vi "Timing.vi"(8 "error in (no error)":errorcluster, 11 "State":T1) -> (0 "error out":errorcluster, 3 "Array":timestamp[](array[timestamp]))   [LabVIEW 2012]
uses:
  New_Framework_2013/State_Machine_Enum.ctl
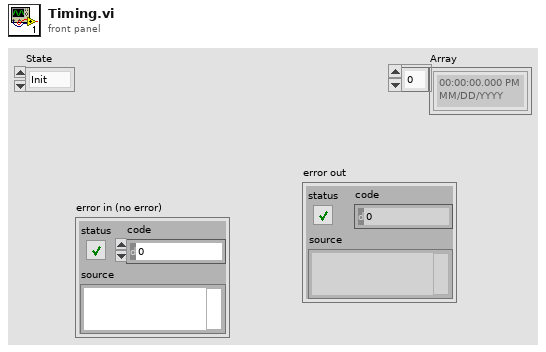
[diagram p1: front panel]
types:
  T1 = typedef "State_Machine_Enum.ctl" = enum16{"Init", "Idle", "Start", "Do", "Stop"}
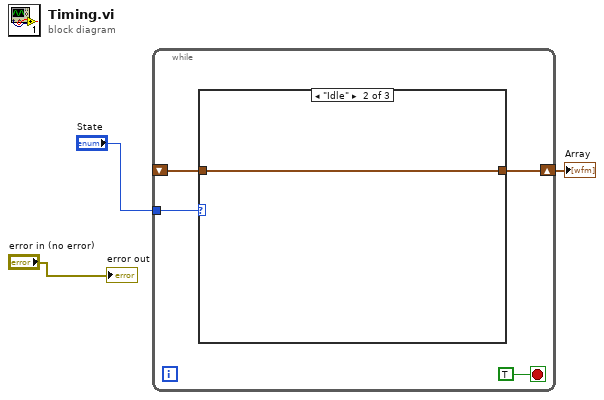
[diagram p0: block diagram]
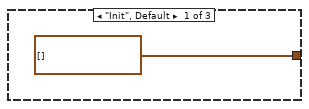
[diagram p2: hidden frame]
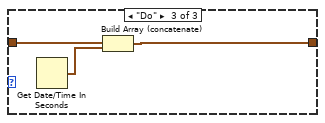
[diagram p3: hidden frame]
diagram:
  n1 = while {
    shift-right: [w7] -> w3
    shift-left: _ -> [w6]
    tunnel: "State" -> [w4]
    stop <- TRUE stop-if-true
    n2 = case shown="\"Idle\"" w4 {
      tunnel: [timestamp[] [] w9 w11] -> w7
      tunnel: w6 -> [_ w9 w12]
      frame "Init", Default {
      }
      frame "Idle" {
      }
      frame "Do" {
        n3 = Get Date/Time In Seconds() -> (seconds since 1Jan1904=w10:timestamp)
        n4 = Build Array (concatenate)(w12, w10) -> (w11:timestamp[])
      }
    }
  }
  "Array" <- w3
  "error out" <- "error in (no error)"
